vi "Frequency_current_field map_MFLI_PK_v4.0_measureXandY.vi"() -> ()   [LabVIEW 2016]
uses:
  <vilib>/Math Plots/2D Math Plots/2D Compass/2D Compass XCtrl/2D Compass.xctl
  <vilib>/Math Plots/2D Math Plots/2D Compass/2D Compass Datatype/2D Compass Datatype.lvclass
  Labview Drivers/MFLI/LabOneLabVIEW-22.02.26577/LabOneLabVIEW-22.02.26577/Zurich Instruments LabOne/Public/Configure/ziSetValueDouble.vi
  <vilib>/Math Plots/2D Math Plots/2D Compass/2D Compass Datatype/Public/Plot Helper (Vector).vi
  Labview Drivers/MFLI/LabOneLabVIEW-22.02.26577/LabOneLabVIEW-22.02.26577/Zurich Instruments LabOne/Public/Configure/ziGetValueDemodSampleEx.vi
  Labview Drivers/MFLI/LabOneLabVIEW-22.02.26577/LabOneLabVIEW-22.02.26577/Zurich Instruments LabOne/Zurich Instruments LabOne.lvlib
panel:
  in  "Measure Second Harmonic Current?":bool=TRUE
  in  "Number averaging (second harmonic)":i32=50
  in  "Autorange ON?":bool
  in  "Measure Second Harmonic Voltage?":bool
  in  "MFLI Current source/Voltage reader":string="DEV3647"
  out "data":dbl[](array[numeric])=[0.38999904300210686, 122.13037074970735, 6.972893577431705e-07, 1.2795166180217325e-05, 6.450568250497636e-11, 0.0, 170.15838700076765, 179.8047672609114, -20.097468935278, 0.0, 70441.803]
  in  "Number averaging (first harmonic)":i32=1
  in  "wait (ms) [Should be > TC]":u32=5000
  out "2D Compass":refnum<class "2D Plot Datatype.lvclass">[](xcontrol)
  in  "Step 3":dbl[](array[numeric])=[0.04, 0.04] min=-3000.0 max=3000.0 format="%.1e"
  in  "To 3":dbl[](array[numeric])=[7.0, -7.0] min=-3000.0 max=3000.0 format="%.1e"
  in  "From 3":dbl[](array[numeric])=[0.0, 0.0] min=-3000.0 max=3000.0 format="%.1e"
  in  "Tab Control":enum32{"Page 1", "Page 2"}(tab)=enum."Page 2"
  out "Iw vs Vw":cluster{dbl, "Field Reading":dbl}[](graph)=[{6.752718621134307e-13, "Field Reading"=6.081816034517228e-09}, {3.9639798477387415e-09, "Field Reading"=6.446162839710732e-08}, {7.973337710224394e-09, "Field Reading"=1.3070822529689762e-07}, {1.1980894320007212e-08, "Field Reading"=2.1301708498159723e-07}, {1.5990904057993272e-08, "Field Reading"=2.8268544133918733e-07}, {1.9996111650797034e-08, "Field Reading"=3.5482236477303006e-07}, {2.400534666117059e-08, "Field Reading"=4.2327567430694e-07}, {2.800722349467468e-08, "Field Reading"=5.024481108748963e-07}, {3.201355214200622e-08, "Field Reading"=5.73207701290961e-07}, {3.602886057924252e-08, "Field Reading"=6.408242032206597e-07}, {4.0029592079284544e-08, "Field Reading"=7.150994635609651e-07}, {4.4043549463955937e-08, "Field Reading"=7.890491387847592e-07}, {4.8050410980351376e-08, "Field Reading"=8.636898236498978e-07}, {5.205405189864272e-08, "Field Reading"=9.359032020670712e-07}, {5.6056170335994144e-08, "Field Reading"=1.0134208250064639e-06}, {6.006110040781738e-08, "Field Reading"=1.0801189896734763e-06}, {6.407650457950991e-08, "Field Reading"=1.157017799271746e-06}, {6.807679850147895e-08, "Field Reading"=1.223571908735428e-06}, {7.21023440572555e-08, "Field Reading"=1.300878249090366e-06}, {7.612142197841778e-08, "Field Reading"=1.3740376616836122e-06}, {8.013380677703043e-08, "Field Reading"=1.4497798169438424e-06}, {8.413258883874902e-08, "Field Reading"=1.5199655499746968e-06}, {8.81468182126121e-08, "Field Reading"=1.5948188164522483e-06}, {9.214947750799019e-08, "Field Reading"=1.6669947570028151e-06}, {9.61591330581471e-08, "Field Reading"=1.7421137383698782e-06}, {1.0016253832106813e-07, "Field Reading"=1.8098314979660362e-06}, {1.0417257692340365e-07, "Field Reading"=1.8855513250381588e-06}, {1.0818369532898691e-07, "Field Reading"=1.9618785093887747e-06}, {1.1218582132451216e-07, "Field Reading"=2.0348711393931705e-06}, {1.1619441564382123e-07, "Field Reading"=2.10788864479139e-06}, {1.2020719866139288e-07, "Field Reading"=2.183351428437738e-06}, {1.2421432089677758e-07, "Field Reading"=2.2548907316702294e-06}, {1.2821366558565993e-07, "Field Reading"=2.3242128448734923e-06}, {1.3222154670961958e-07, "Field Reading"=2.4006507162449404e-06}, {1.3623903792040753e-07, "Field Reading"=2.4756602824151876e-06}, {1.4024313259907697e-07, "Field Reading"=2.552042614165629e-06}, {1.442521785883789e-07, "Field Reading"=2.620144756978161e-06}, {1.4825805446265412e-07, "Field Reading"=2.692379499895667e-06}, {1.5226941875485597e-07, "Field Reading"=2.7663974907389294e-06}, {1.5627669910985748e-07, "Field Reading"=2.839358194975161e-06}, {1.6028888336617344e-07, "Field Reading"=2.911681627856578e-06}, {1.64302772644462e-07, "Field Reading"=2.9888815311636043e-06}, {1.6830688204588808e-07, "Field Reading"=3.057033036041899e-06}, {1.72312249131026e-07, "Field Reading"=3.134796277755431e-06}, {1.7632530452368395e-07, "Field Reading"=3.2066343708058573e-06}, {1.8034298753162188e-07, "Field Reading"=3.2795756506086883e-06}, {1.8433281290203653e-07, "Field Reading"=3.3535223874428235e-06}, {1.8834454582758565e-07, "Field Reading"=3.427737815687775e-06}, {1.923525886788216e-07, "Field Reading"=3.5037940525395852e-06}, {1.9636648414922318e-07, "Field Reading"=3.575940709860304e-06}, {2.003643068727201e-07, "Field Reading"=3.6476811261535922e-06}, {2.0438258512120876e-07, "Field Reading"=3.7191101089781536e-06}, {2.0839002189648273e-07, "Field Reading"=3.795291495640923e-06}, {2.124038020058244e-07, "Field Reading"=3.867976095996228e-06}, {2.164023667169985e-07, "Field Reading"=3.9392937163044255e-06}, {2.2042055698441663e-07, "Field Reading"=4.014886152002913e-06}, {2.2442432876248857e-07, "Field Reading"=4.088888686249118e-06}, {2.284312216677851e-07, "Field Reading"=4.162362043129873e-06}, {2.3244661758681178e-07, "Field Reading"=4.235758863815432e-06}, {2.3644759593726386e-07, "Field Reading"=4.312355387793181e-06}, {2.40459100592141e-07, "Field Reading"=4.3837197112583985e-06}, {2.444529691753868e-07, "Field Reading"=4.457438197792255e-06}, {2.484731479349489e-07, "Field Reading"=4.536782845780873e-06}, {2.524719528533667e-07, "Field Reading"=4.5990035451671585e-06}, {2.5649035151823195e-07, "Field Reading"=4.674219473122293e-06}, {2.6049079932691624e-07, "Field Reading"=4.754493036596978e-06}, {2.645024431202953e-07, "Field Reading"=4.8229123783948095e-06}, {2.685035511024019e-07, "Field Reading"=4.902907714190253e-06}, {2.7250559729734373e-07, "Field Reading"=4.973338061045356e-06}, {2.765088983761033e-07, "Field Reading"=5.0435466472495134e-06}, {2.8052562384174734e-07, "Field Reading"=5.122127663717767e-06}, {2.845332980147583e-07, "Field Reading"=5.1952956260170585e-06}, {2.8853853813904136e-07, "Field Reading"=5.276049411913597e-06}, {2.9255082029007556e-07, "Field Reading"=5.338393085315031e-06}, {2.965589694513312e-07, "Field Reading"=5.414829696556309e-06}, {3.005655236869771e-07, "Field Reading"=5.486743033872425e-06}, {3.0457127604346063e-07, "Field Reading"=5.561439221710705e-06}, {3.0857328583595214e-07, "Field Reading"=5.635709896350234e-06}, {3.125780613188083e-07, "Field Reading"=5.710622154466396e-06}, {3.1657800532807683e-07, "Field Reading"=5.7785483182008366e-06}, {3.205859793496837e-07, "Field Reading"=5.857257666587692e-06}, {3.2459851875999915e-07, "Field Reading"=5.933638774436689e-06}, {3.2861411834016656e-07, "Field Reading"=6.006913317833202e-06}, {3.326041181095403e-07, "Field Reading"=6.083532252465091e-06}, {3.366250625584465e-07, "Field Reading"=6.154442471014648e-06}, {3.406330536788778e-07, "Field Reading"=6.229292535120157e-06}, {3.4463787946499883e-07, "Field Reading"=6.298496219763628e-06}, {3.4864249001668815e-07, "Field Reading"=6.373935145038675e-06}, {3.5266166624564516e-07, "Field Reading"=6.451494387317105e-06}, {3.5666389193853506e-07, "Field Reading"=6.514138102733205e-06}, {3.606647597559832e-07, "Field Reading"=6.593143261943194e-06}, {3.646750692701237e-07, "Field Reading"=6.665398954773506e-06}, {3.686869138293502e-07, "Field Reading"=6.74274312075813e-06}, {3.726946403456541e-07, "Field Reading"=6.813468465941209e-06}, {3.7669898094509526e-07, "Field Reading"=6.8856155861323415e-06}, {3.80713112581362e-07, "Field Reading"=6.966944500326797e-06}, {3.8472237511467064e-07, "Field Reading"=7.042425427008974e-06}, {3.8873229351956887e-07, "Field Reading"=7.1114276716412805e-06}, {3.927256933734159e-07, "Field Reading"=7.187267238196006e-06}, {3.967382699755616e-07, "Field Reading"=7.255760952145238e-06}, {4.007403346966149e-07, "Field Reading"=7.332970273386945e-06}, {4.0474117306471594e-07, "Field Reading"=7.398287477833807e-06}, {4.0876584765236005e-07, "Field Reading"=7.481043329739446e-06}, {4.127782337495444e-07, "Field Reading"=7.561245791041404e-06}, {4.167710748588386e-07, "Field Reading"=7.625287150125578e-06}, {4.207843547855495e-07, "Field Reading"=7.69946278803481e-06}, {4.2478514945557536e-07, "Field Reading"=7.77262746884222e-06}, {4.2880134280692003e-07, "Field Reading"=7.852636002869716e-06}, {4.32792746566576e-07, "Field Reading"=7.920091802554008e-06}, {4.3680613506318253e-07, "Field Reading"=7.99498395075553e-06}, {4.4081431807847446e-07, "Field Reading"=8.073322022266602e-06}, {4.448169330741503e-07, "Field Reading"=8.141452378236027e-06}, {4.488206033855375e-07, "Field Reading"=8.215523961484074e-06}, {4.5283229725978943e-07, "Field Reading"=8.296738126475706e-06}, {4.5684372674779274e-07, "Field Reading"=8.36464717070889e-06}, {4.608385886916715e-07, "Field Reading"=8.435815670392521e-06}, {4.648372028608092e-07, "Field Reading"=8.50960183432341e-06}, {4.688434660258604e-07, "Field Reading"=8.583646136951763e-06}, {4.7284828197185846e-07, "Field Reading"=8.661893728175319e-06}, {4.768439287079396e-07, "Field Reading"=8.736479884477248e-06}, {4.808619754053666e-07, "Field Reading"=8.809133393554074e-06}, {4.848645388187712e-07, "Field Reading"=8.882270213481318e-06}, {4.888608773602841e-07, "Field Reading"=8.957131138329231e-06}, {4.928773928894314e-07, "Field Reading"=9.029727125247536e-06}, {4.9688603946784e-07, "Field Reading"=9.09868256245665e-06}, {5.008984812780072e-07, "Field Reading"=9.179684427963169e-06}, {5.049082694364706e-07, "Field Reading"=9.249396431237732e-06}, {5.089078867339119e-07, "Field Reading"=9.324815631609967e-06}, {5.129207792266292e-07, "Field Reading"=9.395502077706966e-06}, {5.16916821905768e-07, "Field Reading"=9.472861187304162e-06}, {5.209265519237412e-07, "Field Reading"=9.546361127234214e-06}, {5.249452832449703e-07, "Field Reading"=9.618642611519832e-06}, {5.289438730221308e-07, "Field Reading"=9.694146727945345e-06}, {5.329597666740567e-07, "Field Reading"=9.767514041008244e-06}, {5.36959974106049e-07, "Field Reading"=9.839237049373114e-06}, {5.409662739596735e-07, "Field Reading"=9.914717226759983e-06}, {5.449718528352936e-07, "Field Reading"=9.990606585930911e-06}, {5.489786573931961e-07, "Field Reading"=1.0068577997840325e-05}, {5.529795197615837e-07, "Field Reading"=1.0136510865604639e-05}, {5.569935375050876e-07, "Field Reading"=1.0204353143660428e-05}, {5.610099608578356e-07, "Field Reading"=1.0287332733542272e-05}, {5.650150940524591e-07, "Field Reading"=1.0364184451311051e-05}, {5.690251886958287e-07, "Field Reading"=1.0434862772017799e-05}, {5.730169395286551e-07, "Field Reading"=1.0508974657641133e-05}, {5.770317848841414e-07, "Field Reading"=1.058225379853519e-05}, {5.810402693058221e-07, "Field Reading"=1.0643951886158547e-05}, {5.850385166513102e-07, "Field Reading"=1.0725287037518511e-05}, {5.890559617454273e-07, "Field Reading"=1.0803765882597764e-05}, {5.930620244448425e-07, "Field Reading"=1.087588955313183e-05}, {5.970691912424186e-07, "Field Reading"=1.0955708857144528e-05}, {6.010636610044308e-07, "Field Reading"=1.1022087238492938e-05}, {6.050869253358961e-07, "Field Reading"=1.1092486372215814e-05}, {6.09091758211083e-07, "Field Reading"=1.1171170102501748e-05}, {6.131038344649093e-07, "Field Reading"=1.1245702001760147e-05}, {6.171179741498633e-07, "Field Reading"=1.1315855906438373e-05}, {6.211173983599906e-07, "Field Reading"=1.1398578240820748e-05}, {6.25124464451616e-07, "Field Reading"=1.1470196348734225e-05}, {6.291143503695416e-07, "Field Reading"=1.1539420089136223e-05}, {6.331521942370854e-07, "Field Reading"=1.1612792846117975e-05}, {6.371585234008393e-07, "Field Reading"=1.168916434048833e-05}, {6.411653272180744e-07, "Field Reading"=1.1765692996642987e-05}, {6.451832442213258e-07, "Field Reading"=1.1837901362754748e-05}, {6.491850515885537e-07, "Field Reading"=1.1909649783672709e-05}, {6.531930037237445e-07, "Field Reading"=1.198364650491436e-05}, {6.57186432677824e-07, "Field Reading"=1.2060179816420713e-05}, {6.611944104561734e-07, "Field Reading"=1.2123913771082415e-05}, {6.652137445236548e-07, "Field Reading"=1.2211051397225869e-05}, {6.692383358637068e-07, "Field Reading"=1.228412079260952e-05}, {6.732320428385544e-07, "Field Reading"=1.2349533947404962e-05}, {6.77225045428776e-07, "Field Reading"=1.2431989103460716e-05}, {6.812433375195916e-07, "Field Reading"=1.2506056808250104e-05}, {6.852323969852692e-07, "Field Reading"=1.2570407083013278e-05}, {6.892588291001929e-07, "Field Reading"=1.2642367874243355e-05}, {6.932649734064215e-07, "Field Reading"=1.272520742379873e-05}, {6.972796026622005e-07, "Field Reading"=1.2799370686555177e-05}, {3.695457990726968e-13, "Field Reading"=5.698071894479665e-09}, {3.9587514266942006e-09, "Field Reading"=6.824533699184529e-08}, {7.96951312709428e-09, "Field Reading"=1.3985866558682618e-07}, {1.1979948269645202e-08, "Field Reading"=2.0876330521373007e-07}, {1.5983895481099715e-08, "Field Reading"=2.8553830537874887e-07}, {1.999461838939512e-08, "Field Reading"=3.5439162282040604e-07}, {2.400475052994454e-08, "Field Reading"=4.298294578476292e-07}, {2.8008164339990668e-08, "Field Reading"=4.987382728457851e-07}, {3.2017033835969435e-08, "Field Reading"=5.688707826463316e-07}, {3.6024138533788023e-08, "Field Reading"=6.444474335860795e-07}, {4.0033084139702645e-08, "Field Reading"=7.195800417578632e-07}, {4.404046569235817e-08, "Field Reading"=7.927852549096227e-07}, {4.804030826522434e-08, "Field Reading"=8.629720258383935e-07}, {5.2053716184112815e-08, "Field Reading"=9.360625502405603e-07}, {5.605280909327427e-08, "Field Reading"=1.0125975343316225e-06}, {6.006067257344079e-08, "Field Reading"=1.0764321470005743e-06}, {6.406676809702357e-08, "Field Reading"=1.1588846026323697e-06}, {6.807860867321008e-08, "Field Reading"=1.2332259105577365e-06}, {7.210710309990868e-08, "Field Reading"=1.3038192588178447e-06}, {7.61215638566199e-08, "Field Reading"=1.377617098101442e-06}, {8.013214642451544e-08, "Field Reading"=1.452241236858506e-06}, {8.413063130992341e-08, "Field Reading"=1.5205875191624804e-06}, {8.814196552563718e-08, "Field Reading"=1.5973871888974442e-06}, {9.214185329913215e-08, "Field Reading"=1.6636245029512032e-06}, {9.614508769864244e-08, "Field Reading"=1.7505852312657933e-06}, {1.0015602426408757e-07, "Field Reading"=1.8159915918622937e-06}, {1.0416799861410451e-07, "Field Reading"=1.889798444386677e-06}, {1.0817850150530281e-07, "Field Reading"=1.9621860666582506e-06}, {1.1218636839353559e-07, "Field Reading"=2.037082818202477e-06}, {1.1618679588891763e-07, "Field Reading"=2.1122360696148114e-06}, {1.20206814334114e-07, "Field Reading"=2.1777435655423606e-06}, {1.2420841447754306e-07, "Field Reading"=2.255640179281544e-06}, {1.2821319899579289e-07, "Field Reading"=2.3312999651233155e-06}, {1.3222583172501857e-07, "Field Reading"=2.4024085147188928e-06}, {1.3623342017385734e-07, "Field Reading"=2.470034801634953e-06}, {1.4023759008988892e-07, "Field Reading"=2.542095290460891e-06}, {1.4424507010539416e-07, "Field Reading"=2.6170694941540647e-06}, {1.4825488632240412e-07, "Field Reading"=2.6910231312422564e-06}, {1.5226944571136413e-07, "Field Reading"=2.767609787104627e-06}, {1.5627380498979698e-07, "Field Reading"=2.836982731189964e-06}, {1.6028521355674098e-07, "Field Reading"=2.9124222293071654e-06}, {1.6429549429076714e-07, "Field Reading"=2.98472936879348e-06}, {1.6830459853200048e-07, "Field Reading"=3.0613950402695295e-06}, {1.7230366928244657e-07, "Field Reading"=3.1341415581016698e-06}, {1.763177572165781e-07, "Field Reading"=3.2064854067003242e-06}, {1.8032634203251206e-07, "Field Reading"=3.2845130790126582e-06}, {1.843385157463384e-07, "Field Reading"=3.3538281951650226e-06}, {1.883360416878448e-07, "Field Reading"=3.4263295581242788e-06}, {1.9235097490243074e-07, "Field Reading"=3.5074895309486576e-06}, {1.963587115606858e-07, "Field Reading"=3.5723242839209554e-06}, {2.0035576123493957e-07, "Field Reading"=3.6475948759770374e-06}, {2.0437128654225753e-07, "Field Reading"=3.7218891800187525e-06}, {2.0839327750961732e-07, "Field Reading"=3.7922256473378546e-06}, {2.1240028490422649e-07, "Field Reading"=3.872031784491173e-06}, {2.164061391970429e-07, "Field Reading"=3.945420127797786e-06}, {2.204174174016725e-07, "Field Reading"=4.021578337019413e-06}, {2.244213840752897e-07, "Field Reading"=4.092386623889813e-06}, {2.284271593682132e-07, "Field Reading"=4.166951249319548e-06}, {2.3242717177197805e-07, "Field Reading"=4.236549079746125e-06}, {2.364378821769146e-07, "Field Reading"=4.311334792355854e-06}, {2.404587274544687e-07, "Field Reading"=4.388619871276434e-06}, {2.4445827509569344e-07, "Field Reading"=4.458633334353797e-06}, {2.484639539614582e-07, "Field Reading"=4.53699551342188e-06}, {2.5247251325782825e-07, "Field Reading"=4.608124088996196e-06}, {2.564864821249374e-07, "Field Reading"=4.676182220931797e-06}, {2.604810430740118e-07, "Field Reading"=4.749533663063404e-06}, {2.644922890184137e-07, "Field Reading"=4.832174173068287e-06}, {2.685017817576427e-07, "Field Reading"=4.898860317406063e-06}, {2.7250814828756673e-07, "Field Reading"=4.975528351103424e-06}, {2.7651510514395105e-07, "Field Reading"=5.047764978603785e-06}, {2.8052364030662375e-07, "Field Reading"=5.121023562689988e-06}, {2.845325098385667e-07, "Field Reading"=5.191596520538841e-06}, {2.8852780990468735e-07, "Field Reading"=5.266104213036381e-06}, {2.9253698894593535e-07, "Field Reading"=5.339115119283014e-06}, {2.965481465083192e-07, "Field Reading"=5.4160485405172955e-06}, {3.005509495572527e-07, "Field Reading"=5.494915806924091e-06}, {3.045556885916384e-07, "Field Reading"=5.562080696404206e-06}, {3.0856645522803797e-07, "Field Reading"=5.640022217720643e-06}, {3.1257657708335385e-07, "Field Reading"=5.711968405659509e-06}, {3.165750585263558e-07, "Field Reading"=5.783886367669718e-06}, {3.205868903108242e-07, "Field Reading"=5.865148500569075e-06}, {3.2460314250582997e-07, "Field Reading"=5.932597590428266e-06}, {3.2861616400364176e-07, "Field Reading"=6.005949376746854e-06}, {3.3260995873295346e-07, "Field Reading"=6.077729052169175e-06}, {3.3660992509423754e-07, "Field Reading"=6.152365015910243e-06}, {3.406347123545983e-07, "Field Reading"=6.226174256027512e-06}, {3.446438482062892e-07, "Field Reading"=6.299362766035275e-06}, {3.4864186399793596e-07, "Field Reading"=6.37414832191692e-06}, {3.5265247503792236e-07, "Field Reading"=6.4456282419928234e-06}, {3.56665376184869e-07, "Field Reading"=6.529403005613757e-06}, {3.6066734451414065e-07, "Field Reading"=6.598974149679032e-06}, {3.646819848739686e-07, "Field Reading"=6.669921751490827e-06}, {3.68682217504304e-07, "Field Reading"=6.74306226885469e-06}, {3.727065021065556e-07, "Field Reading"=6.813830310377108e-06}, {3.767008614692342e-07, "Field Reading"=6.889393283775725e-06}, {3.807063218593253e-07, "Field Reading"=6.9638747325355745e-06}, {3.84719016492907e-07, "Field Reading"=7.04128753160004e-06}, {3.887276604305829e-07, "Field Reading"=7.105086495008707e-06}, {3.9272401348056196e-07, "Field Reading"=7.184782839715714e-06}, {3.9673291791571813e-07, "Field Reading"=7.256439856497261e-06}, {4.007442843832284e-07, "Field Reading"=7.333113887113307e-06}, {4.0474697892816316e-07, "Field Reading"=7.406217828105429e-06}, {4.0875677214397327e-07, "Field Reading"=7.480073316850151e-06}, {4.127648928978671e-07, "Field Reading"=7.555521781310909e-06}, {4.1677390804238657e-07, "Field Reading"=7.629965109442134e-06}, {4.207784398524056e-07, "Field Reading"=7.699214206031809e-06}, {4.2479118536657584e-07, "Field Reading"=7.777609218528186e-06}, {4.2879348216478443e-07, "Field Reading"=7.848748128930635e-06}, {4.3281368700915934e-07, "Field Reading"=7.927107003998515e-06}, {4.3679043785765377e-07, "Field Reading"=7.991439002710923e-06}, {4.408048794075155e-07, "Field Reading"=8.067457866553554e-06}, {4.4481269705169036e-07, "Field Reading"=8.144639903942311e-06}, {4.488200396041691e-07, "Field Reading"=8.214798069684028e-06}, {4.528261552426099e-07, "Field Reading"=8.288810559972375e-06}, {4.568249367581602e-07, "Field Reading"=8.362134306894896e-06}, {4.6083876371440633e-07, "Field Reading"=8.441314782601667e-06}, {4.6484674569200007e-07, "Field Reading"=8.516255633827248e-06}, {4.6886211987917445e-07, "Field Reading"=8.585900603542732e-06}, {4.728744132518244e-07, "Field Reading"=8.660223005475944e-06}, {4.768710286573309e-07, "Field Reading"=8.734395533820769e-06}, {4.808789492496296e-07, "Field Reading"=8.81077402330044e-06}, {4.84900141033635e-07, "Field Reading"=8.88221335148442e-06}, {4.889096292480101e-07, "Field Reading"=8.952780895721028e-06}, {4.929011448030727e-07, "Field Reading"=9.023233785652485e-06}, {4.96914094104685e-07, "Field Reading"=9.104837016112909e-06}, {5.009124658723474e-07, "Field Reading"=9.176498231786628e-06}, {5.049277646516033e-07, "Field Reading"=9.249998779045577e-06}, {5.089242736925264e-07, "Field Reading"=9.323919830596103e-06}, {5.129328196325962e-07, "Field Reading"=9.393459654395195e-06}, {5.16938938636249e-07, "Field Reading"=9.47134583847599e-06}, {5.209582762725067e-07, "Field Reading"=9.546837597673096e-06}, {5.249599054021532e-07, "Field Reading"=9.618382737867968e-06}, {5.289653219925673e-07, "Field Reading"=9.694529837036145e-06}, {5.329687909235363e-07, "Field Reading"=9.76751027295797e-06}, {5.369619247055903e-07, "Field Reading"=9.844620993541572e-06}, {5.40969967063774e-07, "Field Reading"=9.912999800724708e-06}, {5.449778733989274e-07, "Field Reading"=9.990301579757168e-06}, {5.489887919647749e-07, "Field Reading"=1.0064592865440964e-05}, {5.529916068346236e-07, "Field Reading"=1.0142889568006644e-05}, {5.56988870365852e-07, "Field Reading"=1.021472085789113e-05}, {5.610052420776777e-07, "Field Reading"=1.0289674029122719e-05}, {5.650190658830066e-07, "Field Reading"=1.0360405759120638e-05}, {5.690190702763405e-07, "Field Reading"=1.0435454384407978e-05}, {5.730444454840748e-07, "Field Reading"=1.051298872134457e-05}, {5.770597664108027e-07, "Field Reading"=1.0579031486891604e-05}, {5.810602653692694e-07, "Field Reading"=1.0652944257386492e-05}, {5.850728145256359e-07, "Field Reading"=1.0726243307849132e-05}, {5.890767670181646e-07, "Field Reading"=1.0806947934543218e-05}, {5.930767090913838e-07, "Field Reading"=1.0882796022214024e-05}, {5.970839166377572e-07, "Field Reading"=1.0954573224921726e-05}, {6.011068573945384e-07, "Field Reading"=1.102260076791975e-05}, {6.051002836487515e-07, "Field Reading"=1.1098742423853433e-05}, {6.091153782577642e-07, "Field Reading"=1.1170709784497336e-05}, {6.131153170489284e-07, "Field Reading"=1.1251955700466336e-05}, {6.171206045524325e-07, "Field Reading"=1.1323281210948316e-05}, {6.21125067983006e-07, "Field Reading"=1.1400015059159992e-05}, {6.251268851331833e-07, "Field Reading"=1.1465098896193353e-05}, {6.291438341148671e-07, "Field Reading"=1.1540414658402066e-05}, {6.33130907845599e-07, "Field Reading"=1.1614826739965938e-05}, {6.371470053501204e-07, "Field Reading"=1.1689446616607722e-05}, {6.411561580168332e-07, "Field Reading"=1.1763747227943706e-05}, {6.451858613647945e-07, "Field Reading"=1.1833126732492007e-05}, {6.491750497259894e-07, "Field Reading"=1.1909692915691624e-05}, {6.531963349907788e-07, "Field Reading"=1.198589421633311e-05}, {6.57207107516709e-07, "Field Reading"=1.2059265376888092e-05}, {6.612002662512429e-07, "Field Reading"=1.2131046148000714e-05}, {6.652059118331257e-07, "Field Reading"=1.220693579151733e-05}, {6.692193621767105e-07, "Field Reading"=1.22842018338008e-05}, {6.732075867086699e-07, "Field Reading"=1.2354259434976681e-05}, {6.772319470513882e-07, "Field Reading"=1.242573840875969e-05}, {6.812475180349191e-07, "Field Reading"=1.251079414204885e-05}, {6.852374483111342e-07, "Field Reading"=1.257628484636858e-05}, {6.892677466242672e-07, "Field Reading"=1.2653903437863818e-05}, {6.932781230420922e-07, "Field Reading"=1.2727229374328647e-05}, {6.972893577431705e-07, "Field Reading"=1.2795166180217325e-05}]
  out "I2w (A)":dbl=6.450568250497636e-11
  out "V2w (V)":dbl
  out "Iw (A)":dbl=6.972893577431705e-07
  out "Iw_phase (deg)":dbl=170.15838700076765 format="%#_13g"
  out "Vw (V)":dbl=1.2795166180217325e-05
  out "Vw_phase (deg)":dbl=179.8047672609114 format="%#_13g"
  out "Set Voltage(V)":dbl=-9.84292639411675 format="%#_13g"
  out "Time(s)":dbl=70441.803 format="%#_13g"
  out "I2w_phase (deg)":dbl=-20.097468935278 format="%#_13g"
  out "V2w_phase (deg)":dbl format="%#_13g"
  out "I2w vs Iw":cluster{dbl, "Field Reading":dbl}[](graph)=[{6.752718621134307e-13, "Field Reading"=2.540215775246723e-13}, {3.9639798477387415e-09, "Field Reading"=2.6121334770459845e-12}, {7.973337710224394e-09, "Field Reading"=2.0377945378656124e-12}, {1.1980894320007212e-08, "Field Reading"=2.778071667579133e-12}, {1.5990904057993272e-08, "Field Reading"=2.498846157025503e-12}, {1.9996111650797034e-08, "Field Reading"=1.8837580878055735e-12}, {2.400534666117059e-08, "Field Reading"=2.9217257909799205e-12}, {2.800722349467468e-08, "Field Reading"=1.2408163114046102e-12}, {3.201355214200622e-08, "Field Reading"=1.7629255187333967e-12}, {3.602886057924252e-08, "Field Reading"=2.018708147155936e-12}, {4.0029592079284544e-08, "Field Reading"=7.886162039170557e-13}, {4.4043549463955937e-08, "Field Reading"=2.8246552394199483e-12}, {4.8050410980351376e-08, "Field Reading"=1.2235994978906469e-12}, {5.205405189864272e-08, "Field Reading"=2.644211497717227e-12}, {5.6056170335994144e-08, "Field Reading"=1.3684766141680678e-12}, {6.006110040781738e-08, "Field Reading"=1.1836658755940086e-12}, {6.407650457950991e-08, "Field Reading"=2.235459202881915e-12}, {6.807679850147895e-08, "Field Reading"=9.729688955419961e-13}, {7.21023440572555e-08, "Field Reading"=1.1814396345161887e-11}, {7.612142197841778e-08, "Field Reading"=1.1785466767345847e-11}, {8.013380677703043e-08, "Field Reading"=1.2035102266329501e-11}, {8.413258883874902e-08, "Field Reading"=1.1787630410946756e-11}, {8.81468182126121e-08, "Field Reading"=9.129742332407166e-12}, {9.214947750799019e-08, "Field Reading"=1.033546784505753e-11}, {9.61591330581471e-08, "Field Reading"=1.2123940555621325e-11}, {1.0016253832106813e-07, "Field Reading"=9.689037476398541e-12}, {1.0417257692340365e-07, "Field Reading"=1.080083760883203e-11}, {1.0818369532898691e-07, "Field Reading"=1.2497874907576727e-11}, {1.1218582132451216e-07, "Field Reading"=1.4665030971620474e-11}, {1.1619441564382123e-07, "Field Reading"=1.2342125070206615e-11}, {1.2020719866139288e-07, "Field Reading"=1.616203149927857e-11}, {1.2421432089677758e-07, "Field Reading"=1.2851640441157552e-11}, {1.2821366558565993e-07, "Field Reading"=1.5896882924367085e-11}, {1.3222154670961958e-07, "Field Reading"=1.4119144506488629e-11}, {1.3623903792040753e-07, "Field Reading"=1.250388596871486e-11}, {1.4024313259907697e-07, "Field Reading"=1.4775256013385735e-11}, {1.442521785883789e-07, "Field Reading"=1.4672116340031205e-11}, {1.4825805446265412e-07, "Field Reading"=1.4021899019250218e-11}, {1.5226941875485597e-07, "Field Reading"=1.4698447608535105e-11}, {1.5627669910985748e-07, "Field Reading"=1.4645581087440724e-11}, {1.6028888336617344e-07, "Field Reading"=1.553378665550328e-11}, {1.64302772644462e-07, "Field Reading"=1.4779248598863672e-11}, {1.6830688204588808e-07, "Field Reading"=1.543707856894362e-11}, {1.72312249131026e-07, "Field Reading"=1.519949802066083e-11}, {1.7632530452368395e-07, "Field Reading"=1.5743715585473236e-11}, {1.8034298753162188e-07, "Field Reading"=1.4207409174203727e-11}, {1.8433281290203653e-07, "Field Reading"=1.6044432054311044e-11}, {1.8834454582758565e-07, "Field Reading"=1.6002816819122775e-11}, {1.923525886788216e-07, "Field Reading"=2.0174419803341724e-11}, {1.9636648414922318e-07, "Field Reading"=2.059968665438357e-11}, {2.003643068727201e-07, "Field Reading"=2.016164350039611e-11}, {2.0438258512120876e-07, "Field Reading"=2.3667687802935574e-11}, {2.0839002189648273e-07, "Field Reading"=2.1856416542193945e-11}, {2.124038020058244e-07, "Field Reading"=2.5654034396396907e-11}, {2.164023667169985e-07, "Field Reading"=2.2994401791125607e-11}, {2.2042055698441663e-07, "Field Reading"=2.266592088694829e-11}, {2.2442432876248857e-07, "Field Reading"=2.440238662218269e-11}, {2.284312216677851e-07, "Field Reading"=2.5566886630157963e-11}, {2.3244661758681178e-07, "Field Reading"=2.890025645099675e-11}, {2.3644759593726386e-07, "Field Reading"=2.8182570348539977e-11}, {2.40459100592141e-07, "Field Reading"=2.928977666771924e-11}, {2.444529691753868e-07, "Field Reading"=3.066958341298326e-11}, {2.484731479349489e-07, "Field Reading"=3.209625154731619e-11}, {2.524719528533667e-07, "Field Reading"=3.264451552248229e-11}, {2.5649035151823195e-07, "Field Reading"=3.318956535231248e-11}, {2.6049079932691624e-07, "Field Reading"=3.37335010932016e-11}, {2.645024431202953e-07, "Field Reading"=3.0763102231648744e-11}, {2.685035511024019e-07, "Field Reading"=3.418658009474822e-11}, {2.7250559729734373e-07, "Field Reading"=3.5796418085787905e-11}, {2.765088983761033e-07, "Field Reading"=3.4815474973541285e-11}, {2.8052562384174734e-07, "Field Reading"=3.6164532600325935e-11}, {2.845332980147583e-07, "Field Reading"=3.967574463601413e-11}, {2.8853853813904136e-07, "Field Reading"=4.1219209656416e-11}, {2.9255082029007556e-07, "Field Reading"=4.095310840833821e-11}, {2.965589694513312e-07, "Field Reading"=4.0410146332783684e-11}, {3.005655236869771e-07, "Field Reading"=3.820479698209618e-11}, {3.0457127604346063e-07, "Field Reading"=4.2137836009754024e-11}, {3.0857328583595214e-07, "Field Reading"=3.9451625172654855e-11}, {3.125780613188083e-07, "Field Reading"=4.2371481330199476e-11}, {3.1657800532807683e-07, "Field Reading"=3.8881852757914235e-11}, {3.205859793496837e-07, "Field Reading"=3.771658107955753e-11}, {3.2459851875999915e-07, "Field Reading"=4.156223942591132e-11}, {3.2861411834016656e-07, "Field Reading"=3.729691749797255e-11}, {3.326041181095403e-07, "Field Reading"=3.818853589427644e-11}, {3.366250625584465e-07, "Field Reading"=3.867563543286446e-11}, {3.406330536788778e-07, "Field Reading"=4.0896864114161576e-11}, {3.4463787946499883e-07, "Field Reading"=4.049615787642101e-11}, {3.4864249001668815e-07, "Field Reading"=4.109707653892744e-11}, {3.5266166624564516e-07, "Field Reading"=3.6936103946973474e-11}, {3.5666389193853506e-07, "Field Reading"=3.9768558666395626e-11}, {3.606647597559832e-07, "Field Reading"=3.972307596471419e-11}, {3.646750692701237e-07, "Field Reading"=4.3807969619634275e-11}, {3.686869138293502e-07, "Field Reading"=4.241465760875651e-11}, {3.726946403456541e-07, "Field Reading"=4.333193505611894e-11}, {3.7669898094509526e-07, "Field Reading"=4.395923375273165e-11}, {3.80713112581362e-07, "Field Reading"=4.1158201011650476e-11}, {3.8472237511467064e-07, "Field Reading"=4.599634818218701e-11}, {3.8873229351956887e-07, "Field Reading"=4.4910724411118646e-11}, {3.927256933734159e-07, "Field Reading"=4.442976934059301e-11}, {3.967382699755616e-07, "Field Reading"=4.1494924497488085e-11}, {4.007403346966149e-07, "Field Reading"=4.327928671432316e-11}, {4.0474117306471594e-07, "Field Reading"=4.446850731516231e-11}, {4.0876584765236005e-07, "Field Reading"=4.7651102924287676e-11}, {4.127782337495444e-07, "Field Reading"=4.723442322285639e-11}, {4.167710748588386e-07, "Field Reading"=4.806634095914595e-11}, {4.207843547855495e-07, "Field Reading"=4.86904396373397e-11}, {4.2478514945557536e-07, "Field Reading"=4.941079980687742e-11}, {4.2880134280692003e-07, "Field Reading"=5.1576537234183364e-11}, {4.32792746566576e-07, "Field Reading"=5.0784095230428863e-11}, {4.3680613506318253e-07, "Field Reading"=5.3128892662127496e-11}, {4.4081431807847446e-07, "Field Reading"=5.155216721523001e-11}, {4.448169330741503e-07, "Field Reading"=5.105613828796419e-11}, {4.488206033855375e-07, "Field Reading"=5.226617929286254e-11}, {4.5283229725978943e-07, "Field Reading"=5.230436353459349e-11}, {4.5684372674779274e-07, "Field Reading"=5.050267037525422e-11}, {4.608385886916715e-07, "Field Reading"=4.84499271575798e-11}, {4.648372028608092e-07, "Field Reading"=5.0190924304783066e-11}, {4.688434660258604e-07, "Field Reading"=4.8448919752355426e-11}, {4.7284828197185846e-07, "Field Reading"=5.0993456513791535e-11}, {4.768439287079396e-07, "Field Reading"=5.017036670880965e-11}, {4.808619754053666e-07, "Field Reading"=5.325372655862345e-11}, {4.848645388187712e-07, "Field Reading"=5.3656986374214387e-11}, {4.888608773602841e-07, "Field Reading"=5.415062023945687e-11}, {4.928773928894314e-07, "Field Reading"=5.125431277495083e-11}, {4.9688603946784e-07, "Field Reading"=5.20620903173094e-11}, {5.008984812780072e-07, "Field Reading"=5.200329148338377e-11}, {5.049082694364706e-07, "Field Reading"=5.5944855456576576e-11}, {5.089078867339119e-07, "Field Reading"=5.559808794958296e-11}, {5.129207792266292e-07, "Field Reading"=5.3286662644534903e-11}, {5.16916821905768e-07, "Field Reading"=5.498606317557074e-11}, {5.209265519237412e-07, "Field Reading"=5.271909693376304e-11}, {5.249452832449703e-07, "Field Reading"=5.5509562837912806e-11}, {5.289438730221308e-07, "Field Reading"=5.4232980137627814e-11}, {5.329597666740567e-07, "Field Reading"=5.546771331901801e-11}, {5.36959974106049e-07, "Field Reading"=5.247671999342142e-11}, {5.409662739596735e-07, "Field Reading"=5.350919505243116e-11}, {5.449718528352936e-07, "Field Reading"=5.507408335848158e-11}, {5.489786573931961e-07, "Field Reading"=5.394514289016507e-11}, {5.529795197615837e-07, "Field Reading"=5.416509011512546e-11}, {5.569935375050876e-07, "Field Reading"=5.73465618608679e-11}, {5.610099608578356e-07, "Field Reading"=5.930803544847915e-11}, {5.650150940524591e-07, "Field Reading"=6.005414940478683e-11}, {5.690251886958287e-07, "Field Reading"=5.888737721954652e-11}, {5.730169395286551e-07, "Field Reading"=6.077411503763882e-11}, {5.770317848841414e-07, "Field Reading"=6.107877071768294e-11}, {5.810402693058221e-07, "Field Reading"=5.900724881515841e-11}, {5.850385166513102e-07, "Field Reading"=6.006440069880428e-11}, {5.890559617454273e-07, "Field Reading"=5.91486657994636e-11}, {5.930620244448425e-07, "Field Reading"=6.200190538257744e-11}, {5.970691912424186e-07, "Field Reading"=6.376389691530029e-11}, {6.010636610044308e-07, "Field Reading"=6.568419928169567e-11}, {6.050869253358961e-07, "Field Reading"=6.646824219614154e-11}, {6.09091758211083e-07, "Field Reading"=6.562652637844236e-11}, {6.131038344649093e-07, "Field Reading"=6.43058326727766e-11}, {6.171179741498633e-07, "Field Reading"=6.568558396814543e-11}, {6.211173983599906e-07, "Field Reading"=6.768436991877683e-11}, {6.25124464451616e-07, "Field Reading"=6.756103006652947e-11}, {6.291143503695416e-07, "Field Reading"=6.820302809524011e-11}, {6.331521942370854e-07, "Field Reading"=6.694996980417711e-11}, {6.371585234008393e-07, "Field Reading"=6.519799519752896e-11}, {6.411653272180744e-07, "Field Reading"=6.613374278434862e-11}, {6.451832442213258e-07, "Field Reading"=6.796003831239519e-11}, {6.491850515885537e-07, "Field Reading"=6.710962755139632e-11}, {6.531930037237445e-07, "Field Reading"=6.734378786394395e-11}, {6.57186432677824e-07, "Field Reading"=6.677330526833857e-11}, {6.611944104561734e-07, "Field Reading"=6.674662242254714e-11}, {6.652137445236548e-07, "Field Reading"=6.951367305557199e-11}, {6.692383358637068e-07, "Field Reading"=7.056981059966933e-11}, {6.732320428385544e-07, "Field Reading"=7.013612722864493e-11}, {6.77225045428776e-07, "Field Reading"=7.016545459975179e-11}, {6.812433375195916e-07, "Field Reading"=6.871880309362113e-11}, {6.852323969852692e-07, "Field Reading"=6.829047114108872e-11}, {6.892588291001929e-07, "Field Reading"=6.483165357707174e-11}, {6.932649734064215e-07, "Field Reading"=6.490006655716477e-11}, {6.972796026622005e-07, "Field Reading"=6.422401070609759e-11}, {3.695457990726968e-13, "Field Reading"=2.5282771557741105e-13}, {3.9587514266942006e-09, "Field Reading"=1.5930535501026506e-12}, {7.96951312709428e-09, "Field Reading"=2.8010787419509677e-12}, {1.1979948269645202e-08, "Field Reading"=2.013426834849837e-12}, {1.5983895481099715e-08, "Field Reading"=1.829543393434864e-12}, {1.999461838939512e-08, "Field Reading"=3.066066372911442e-12}, {2.400475052994454e-08, "Field Reading"=1.5706011088297255e-12}, {2.8008164339990668e-08, "Field Reading"=3.6665461606118e-12}, {3.2017033835969435e-08, "Field Reading"=2.237745011419964e-12}, {3.6024138533788023e-08, "Field Reading"=1.1721437631620448e-12}, {4.0033084139702645e-08, "Field Reading"=2.0262995104221244e-12}, {4.404046569235817e-08, "Field Reading"=3.664943475534297e-12}, {4.804030826522434e-08, "Field Reading"=2.263797066505037e-12}, {5.2053716184112815e-08, "Field Reading"=2.620818120649302e-12}, {5.605280909327427e-08, "Field Reading"=2.318384645557775e-12}, {6.006067257344079e-08, "Field Reading"=1.9418907259098453e-12}, {6.406676809702357e-08, "Field Reading"=2.531394132444377e-12}, {6.807860867321008e-08, "Field Reading"=1.567379129176001e-12}, {7.210710309990868e-08, "Field Reading"=1.0071141601975999e-11}, {7.61215638566199e-08, "Field Reading"=9.7246564671276e-12}, {8.013214642451544e-08, "Field Reading"=8.901859561486112e-12}, {8.413063130992341e-08, "Field Reading"=8.694430732977649e-12}, {8.814196552563718e-08, "Field Reading"=1.2309012341618928e-11}, {9.214185329913215e-08, "Field Reading"=1.2771534835221438e-11}, {9.614508769864244e-08, "Field Reading"=1.3247622019980793e-11}, {1.0015602426408757e-07, "Field Reading"=1.1623885984399354e-11}, {1.0416799861410451e-07, "Field Reading"=1.0960532276840816e-11}, {1.0817850150530281e-07, "Field Reading"=1.177907035266872e-11}, {1.1218636839353559e-07, "Field Reading"=1.4879678755840352e-11}, {1.1618679588891763e-07, "Field Reading"=1.5184060031636686e-11}, {1.20206814334114e-07, "Field Reading"=1.4358689089879189e-11}, {1.2420841447754306e-07, "Field Reading"=1.6463444299038886e-11}, {1.2821319899579289e-07, "Field Reading"=1.3332194594148655e-11}, {1.3222583172501857e-07, "Field Reading"=1.691280787353132e-11}, {1.3623342017385734e-07, "Field Reading"=1.478275840209281e-11}, {1.4023759008988892e-07, "Field Reading"=1.424375001618506e-11}, {1.4424507010539416e-07, "Field Reading"=1.4256112803461382e-11}, {1.4825488632240412e-07, "Field Reading"=1.4333770233563216e-11}, {1.5226944571136413e-07, "Field Reading"=1.2888064058912636e-11}, {1.5627380498979698e-07, "Field Reading"=1.0486184893392225e-11}, {1.6028521355674098e-07, "Field Reading"=1.1700279364616469e-11}, {1.6429549429076714e-07, "Field Reading"=1.0998345543133605e-11}, {1.6830459853200048e-07, "Field Reading"=1.2087743463677898e-11}, {1.7230366928244657e-07, "Field Reading"=1.3471449267382825e-11}, {1.763177572165781e-07, "Field Reading"=1.608972699679182e-11}, {1.8032634203251206e-07, "Field Reading"=1.7305910558522267e-11}, {1.843385157463384e-07, "Field Reading"=1.8368738005846515e-11}, {1.883360416878448e-07, "Field Reading"=1.9289506796775354e-11}, {1.9235097490243074e-07, "Field Reading"=1.9779973910331214e-11}, {1.963587115606858e-07, "Field Reading"=1.8126979945707045e-11}, {2.0035576123493957e-07, "Field Reading"=2.1452009833031672e-11}, {2.0437128654225753e-07, "Field Reading"=2.2998721643182e-11}, {2.0839327750961732e-07, "Field Reading"=2.1212307651756744e-11}, {2.1240028490422649e-07, "Field Reading"=2.2875441587449862e-11}, {2.164061391970429e-07, "Field Reading"=2.3773098810818826e-11}, {2.204174174016725e-07, "Field Reading"=2.7512188257361405e-11}, {2.244213840752897e-07, "Field Reading"=2.3892096852057306e-11}, {2.284271593682132e-07, "Field Reading"=2.699449181851823e-11}, {2.3242717177197805e-07, "Field Reading"=2.909431702211742e-11}, {2.364378821769146e-07, "Field Reading"=2.8973407441934445e-11}, {2.404587274544687e-07, "Field Reading"=2.7884583200848478e-11}, {2.4445827509569344e-07, "Field Reading"=3.027143193005267e-11}, {2.484639539614582e-07, "Field Reading"=3.1564504304575715e-11}, {2.5247251325782825e-07, "Field Reading"=2.9237575937923634e-11}, {2.564864821249374e-07, "Field Reading"=3.053670669953717e-11}, {2.604810430740118e-07, "Field Reading"=3.202430697005556e-11}, {2.644922890184137e-07, "Field Reading"=3.46554090746098e-11}, {2.685017817576427e-07, "Field Reading"=3.578845693699961e-11}, {2.7250814828756673e-07, "Field Reading"=3.7647775293476866e-11}, {2.7651510514395105e-07, "Field Reading"=3.5647085806780566e-11}, {2.8052364030662375e-07, "Field Reading"=3.656104758307045e-11}, {2.845325098385667e-07, "Field Reading"=3.813337986367964e-11}, {2.8852780990468735e-07, "Field Reading"=3.787286335856111e-11}, {2.9253698894593535e-07, "Field Reading"=3.824108014196267e-11}, {2.965481465083192e-07, "Field Reading"=4.132073204569839e-11}, {3.005509495572527e-07, "Field Reading"=4.2408680649944874e-11}, {3.045556885916384e-07, "Field Reading"=4.043608416368307e-11}, {3.0856645522803797e-07, "Field Reading"=4.378766502806668e-11}, {3.1257657708335385e-07, "Field Reading"=4.23446865354141e-11}, {3.165750585263558e-07, "Field Reading"=4.084687863264775e-11}, {3.205868903108242e-07, "Field Reading"=3.77712019884902e-11}, {3.2460314250582997e-07, "Field Reading"=3.8839688695298754e-11}, {3.2861616400364176e-07, "Field Reading"=3.9055940958325796e-11}, {3.3260995873295346e-07, "Field Reading"=4.136158645127124e-11}, {3.3660992509423754e-07, "Field Reading"=3.9915508760910296e-11}, {3.406347123545983e-07, "Field Reading"=4.125702084595111e-11}, {3.446438482062892e-07, "Field Reading"=4.074788836784656e-11}, {3.4864186399793596e-07, "Field Reading"=4.094992368976711e-11}, {3.5265247503792236e-07, "Field Reading"=3.868708943255324e-11}, {3.56665376184869e-07, "Field Reading"=4.103221476082204e-11}, {3.6066734451414065e-07, "Field Reading"=4.1234657494615655e-11}, {3.646819848739686e-07, "Field Reading"=4.260268639569677e-11}, {3.68682217504304e-07, "Field Reading"=4.240946718456471e-11}, {3.727065021065556e-07, "Field Reading"=4.3519965995171096e-11}, {3.767008614692342e-07, "Field Reading"=4.312434943636139e-11}, {3.807063218593253e-07, "Field Reading"=4.3130546030337724e-11}, {3.84719016492907e-07, "Field Reading"=4.008661675930759e-11}, {3.887276604305829e-07, "Field Reading"=4.221198007949393e-11}, {3.9272401348056196e-07, "Field Reading"=4.293936651182658e-11}, {3.9673291791571813e-07, "Field Reading"=4.623167191553964e-11}, {4.007442843832284e-07, "Field Reading"=4.5708175331670406e-11}, {4.0474697892816316e-07, "Field Reading"=4.6507344105935516e-11}, {4.0875677214397327e-07, "Field Reading"=4.6580875212270724e-11}, {4.127648928978671e-07, "Field Reading"=4.535138996722086e-11}, {4.1677390804238657e-07, "Field Reading"=4.5671496639393876e-11}, {4.207784398524056e-07, "Field Reading"=4.5770496014952985e-11}, {4.2479118536657584e-07, "Field Reading"=4.609142706204921e-11}, {4.2879348216478443e-07, "Field Reading"=4.733321843144122e-11}, {4.3281368700915934e-07, "Field Reading"=5.131715035553229e-11}, {4.3679043785765377e-07, "Field Reading"=5.323776363782982e-11}, {4.408048794075155e-07, "Field Reading"=5.20746578553526e-11}, {4.4481269705169036e-07, "Field Reading"=5.094516991074002e-11}, {4.488200396041691e-07, "Field Reading"=5.124597491329243e-11}, {4.528261552426099e-07, "Field Reading"=5.0694648259650356e-11}, {4.568249367581602e-07, "Field Reading"=5.21182348591489e-11}, {4.6083876371440633e-07, "Field Reading"=5.264139350935497e-11}, {4.6484674569200007e-07, "Field Reading"=4.984891293279687e-11}, {4.6886211987917445e-07, "Field Reading"=5.200959708629815e-11}, {4.728744132518244e-07, "Field Reading"=5.2887129747821636e-11}, {4.768710286573309e-07, "Field Reading"=5.3139990203683924e-11}, {4.808789492496296e-07, "Field Reading"=5.274328640383689e-11}, {4.84900141033635e-07, "Field Reading"=5.10394187848172e-11}, {4.889096292480101e-07, "Field Reading"=5.116674902217948e-11}, {4.929011448030727e-07, "Field Reading"=5.129311458492361e-11}, {4.96914094104685e-07, "Field Reading"=5.453118140549034e-11}, {5.009124658723474e-07, "Field Reading"=5.5317619441512025e-11}, {5.049277646516033e-07, "Field Reading"=5.4160712141388186e-11}, {5.089242736925264e-07, "Field Reading"=5.254562653859669e-11}, {5.129328196325962e-07, "Field Reading"=5.0589330539100945e-11}, {5.16938938636249e-07, "Field Reading"=5.403132441467029e-11}, {5.209582762725067e-07, "Field Reading"=5.161295249804235e-11}, {5.249599054021532e-07, "Field Reading"=5.140484581442028e-11}, {5.289653219925673e-07, "Field Reading"=5.310231597481294e-11}, {5.329687909235363e-07, "Field Reading"=5.6550392801717196e-11}, {5.369619247055903e-07, "Field Reading"=5.5442567728589046e-11}, {5.40969967063774e-07, "Field Reading"=5.496185734017828e-11}, {5.449778733989274e-07, "Field Reading"=5.746765226674961e-11}, {5.489887919647749e-07, "Field Reading"=5.7391109065635136e-11}, {5.529916068346236e-07, "Field Reading"=5.8103278479543546e-11}, {5.56988870365852e-07, "Field Reading"=5.765234035640036e-11}, {5.610052420776777e-07, "Field Reading"=5.760578045335417e-11}, {5.650190658830066e-07, "Field Reading"=5.583399297292977e-11}, {5.690190702763405e-07, "Field Reading"=5.7413386199988124e-11}, {5.730444454840748e-07, "Field Reading"=5.965623799055868e-11}, {5.770597664108027e-07, "Field Reading"=5.803920845830859e-11}, {5.810602653692694e-07, "Field Reading"=5.866732708139203e-11}, {5.850728145256359e-07, "Field Reading"=6.220428671391128e-11}, {5.890767670181646e-07, "Field Reading"=6.28457191652954e-11}, {5.930767090913838e-07, "Field Reading"=6.246047345077204e-11}, {5.970839166377572e-07, "Field Reading"=6.477595792134802e-11}, {6.011068573945384e-07, "Field Reading"=6.46726343069814e-11}, {6.051002836487515e-07, "Field Reading"=6.381069130657024e-11}, {6.091153782577642e-07, "Field Reading"=6.155997746024924e-11}, {6.131153170489284e-07, "Field Reading"=6.378432601235624e-11}, {6.171206045524325e-07, "Field Reading"=6.539002976056167e-11}, {6.21125067983006e-07, "Field Reading"=6.748621349202427e-11}, {6.251268851331833e-07, "Field Reading"=6.784349375094177e-11}, {6.291438341148671e-07, "Field Reading"=6.728069780676202e-11}, {6.33130907845599e-07, "Field Reading"=6.671980944956575e-11}, {6.371470053501204e-07, "Field Reading"=6.853978819520523e-11}, {6.411561580168332e-07, "Field Reading"=6.679258842188276e-11}, {6.451858613647945e-07, "Field Reading"=6.615636376498311e-11}, {6.491750497259894e-07, "Field Reading"=6.894322854010631e-11}, {6.531963349907788e-07, "Field Reading"=6.683473570332554e-11}, {6.57207107516709e-07, "Field Reading"=6.70014765968252e-11}, {6.612002662512429e-07, "Field Reading"=6.810761036318809e-11}, {6.652059118331257e-07, "Field Reading"=6.713753432347388e-11}, {6.692193621767105e-07, "Field Reading"=6.625772619668147e-11}, {6.732075867086699e-07, "Field Reading"=6.884905694478715e-11}, {6.772319470513882e-07, "Field Reading"=6.841461144489658e-11}, {6.812475180349191e-07, "Field Reading"=6.522473456669023e-11}, {6.852374483111342e-07, "Field Reading"=6.933465888948014e-11}, {6.892677466242672e-07, "Field Reading"=6.664557132943735e-11}, {6.932781230420922e-07, "Field Reading"=6.565116809569013e-11}, {6.972893577431705e-07, "Field Reading"=6.450568250497636e-11}]
  out "Magnetic Field Vector Angle":dbl=122.13037074970735 format="%#_13g"
  out "Magnetic Field Vector magnitude (T)":dbl=0.38999904300210686 format="%#_13g"
  in  "From 2":dbl[](array[numeric])=[0.15] min=-3000.0 max=3000.0 format="%#.5f"
  in  "To 2":dbl[](array[numeric])=[0.4] min=-3000.0 max=3000.0 format="%#.5g"
  in  "Step 2":dbl[](array[numeric])=[0.01] min=-3000.0 max=3000.0 format="%.3g"
  in  "Wait time after each sweep(min)":dbl format="%#_13g"
  out "Z-axis Magnetic Field (T)":string="0.330266838\r\n"
  in  "Y-axis Field ramp rate (T/min)":string="0.005"
  in  "Z-axis Field ramp rate (T/min)":string="0.005"
  out "Z-axis (90 deg)":dbl(slide)=0.330266838 scale=0.0..3.0
  out "Y-Axis (0deg)":dbl(slide)=-0.207420031 scale=0.0..3.0
  out "Y-axis Magnetic Field (T)":string="-0.207420031\r\n"
  in  "Magnet IP Address Z-axis":string="169.254.134.245"
  in  "Magnet IP Address Y-axis":string="169.254.212.113"
  in  "Magnetic field stabilization time (s)":dbl=2.0 format="%#_13g"
  in  "Step":dbl[](array[numeric])=[0.1] min=-3000.0 max=3000.0 format="%.4g"
  in  "To":dbl[](array[numeric])=[122.13] min=-3000.0 max=3000.0 format="%.4f"
  in  "From":dbl[](array[numeric])=[122.13] min=-3000.0 max=3000.0 format="%.4f"
  in  "Folder":path=path "D:/Pranava/Data/NiTe2/20-01-2021"
  in  "File name":string="006_NiTe2_13-12-2021_001_DeviceB_I_31-33_V_30-35_AC_IV(H)_with_second_harmonic_current_10Mohmbuffer_7.919Hz_7mK_150-400mT_122.13deg(perpendicular_to_current)_50ave_float"
  out "File path":path=path "D:/Pranava/Data/NiTe2/20-01-2021/006_NiTe2_13-12-2021_001_DeviceB_I_31-33_V_30-35_AC_IV(H)_with_second_harmonic_current_10Mohmbuffer_7.919Hz_7mK_150-400mT_122.13deg(perpendicular_to_current)_50ave_float.dat"
  # "Z-Axis: In-plane (90 deg)\nY-axis: Out-of-plane (0 deg)"
  # "[Must be less than 0.05]"
  # ".dat"
  # "It is important that there is enough time for the magnet to cool down after each sweep (Typically 15-20 min)"
  # "Configure Field magnitude (T)"
  # "Configure Field Angle (deg)"
  # "Configure MFLI voltage output (V)"
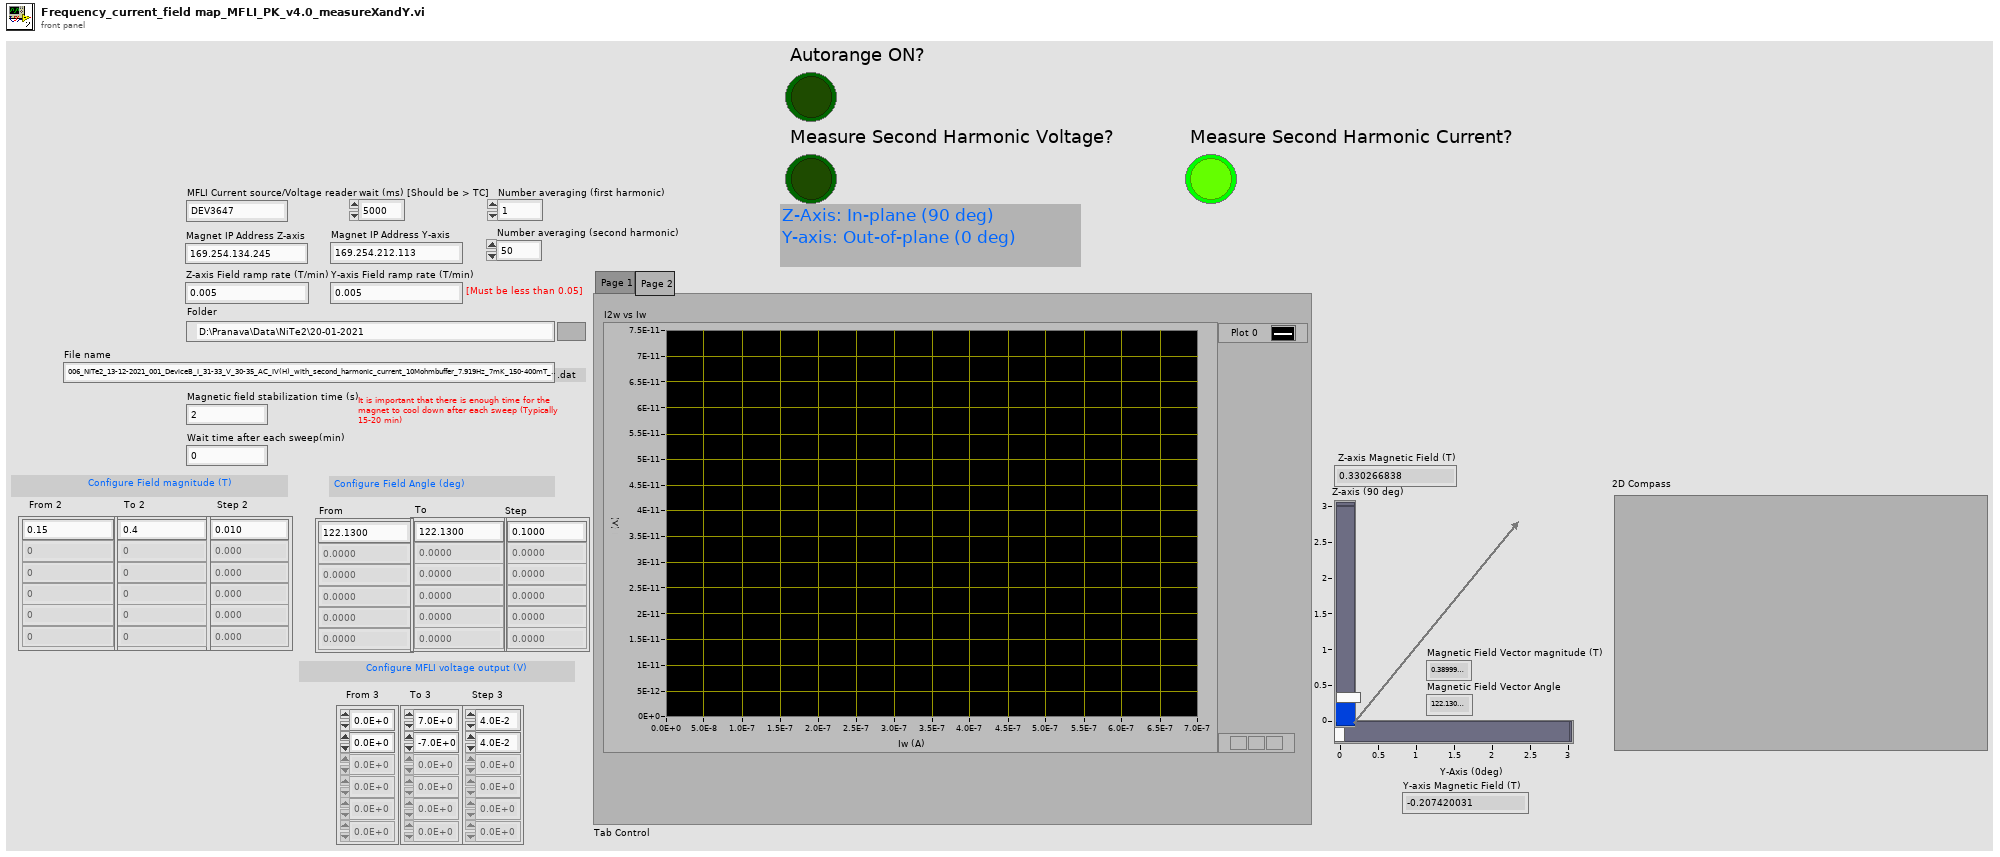
[diagram p1: front panel]
types:
  T1 = typedef "Zurich Instruments LabOne.lvlib/ziTypeHandle.ctl" = cluster{"handleValid":bool, "Conn":u64, "Path Prefix":string, "Handle":u64, "Connected":bool, "Clockbase(s)":dbl}
  T2 = enum16{"open", "replace", "create", "open or create", "replace or create", "replace or create with confirmation"}
  T3 = typedef "Zurich Instruments LabOne.lvlib/ziTypeDemodSampleSingle.ctl" = cluster{"Timestamps (ticks)":u64, "X (Vrms)":dbl, "Y (Vrms)":dbl, "Osc Phase (deg)":dbl, "Freq (Hz)":dbl, "DIO":u32, "AuxIn0 (V)":dbl, "AuxIn1 (V)":dbl, "Trigger":u32}
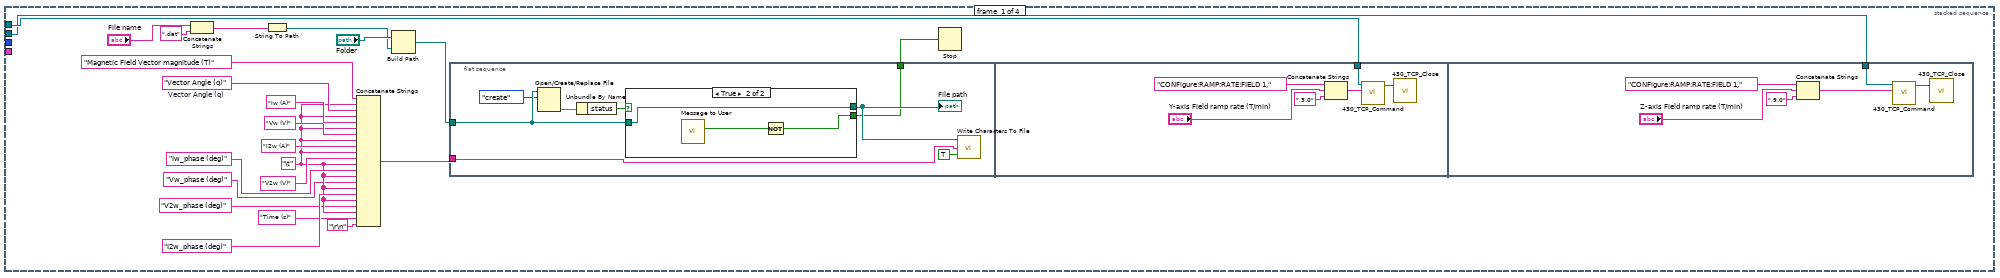
[diagram p2: hidden frame]
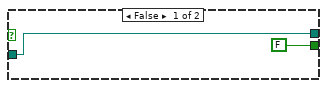
[diagram p3: hidden frame]
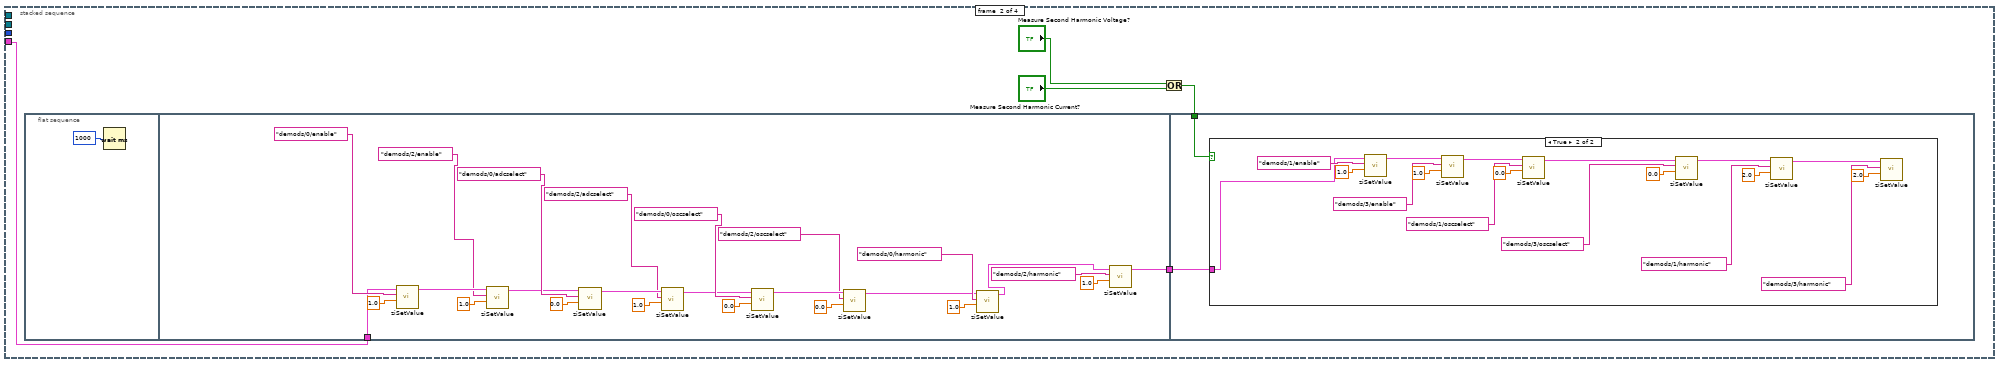
[diagram p4: hidden frame]
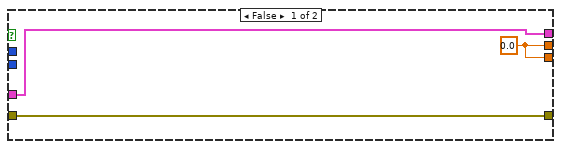
[diagram p8: hidden frame]
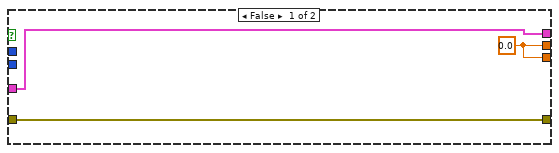
[diagram p9: hidden frame]
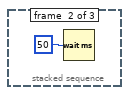
[diagram p10: hidden frame]
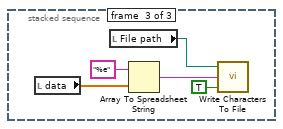
[diagram p11: hidden frame]
diagram:
  n1 = call "ziOpen.vi"("Address"="MFLI Current source/Voltage reader") -> ("Error Out"=w4:errorcluster, "HandleOut"=w5:T1)  [unwired: 3 in, 1 out]
  n2 = call "ziCheckVersion.vi"("Handle In"=w5, "Error In"=w4) -> ("Handle Out"=w2:T1)  [unwired: 11 in, 2 out]
  n3 = call "430_TCP_Open.vi"("IP Address"="Magnet IP Address Y-axis", "TCP Port"=7180) -> ("connection ID"=w11:refnum<k5>)  [unwired: 4 in, 2 out]
  n4 = call "430_TCP_Open.vi"("IP Address"="Magnet IP Address Z-axis", "TCP Port"=7180) -> ("connection ID"=w6:refnum<k5>)  [unwired: 4 in, 2 out]
  n5 = Tick Count (ms)() -> (millisecond timer value=w10:u32)
  n6 = stacked-sequence {
    tunnel: w11 -> [w26 _ _ _]
    tunnel: w10 -> [_ _ w117 _]
    tunnel: w6 -> [w24 _ _ _]
    tunnel: w2 -> [_ w65 w113 _]
    tunnel: [_ _ w112 _] -> w1
    frame #0 {
      w23 = "Vector Angle (q)"  # Vector Angle (q)
      w16 = "\t"
      n7 = Concatenate Strings("File name", ".dat" ("string")) -> (w33:string)
      n8 = String To Path(string=w33) -> (path=w28:path)
      n9 = Concatenate Strings("Magnetic Field Vector magnitude (T)", w16, w23, w16, "Iw (A)" ("string"), w16, "Vw (V)" ("string"), w16, "I2w (A)" ("string"), w16, "V2w (V)" ("string"), w16, "Iw_phase (deg)", w16, "Vw_phase (deg)", w16, "I2w_phase (deg)", w16, "V2w_phase (deg)", w16, "Time (s)", "\r\n") -> (w34:string)
      n10 = Build Path(base path="Folder", name or relative path=w28) -> (appended path=w27:path)
      n11 = flat-sequence {
        tunnel: [w40] -> w31
        tunnel: w34 -> [w42]
        tunnel: w27 -> [w39]
        tunnel: w26 -> [w50]
        tunnel: w24 -> [w55]
        frame #0 {
          n12 = Open/Create/Replace File(file path (use dialog)=w39, operation (0:open)=T2."create") -> (error out=w38:errorcluster)  [unwired: 4 in, 2 out]
          n13 = Unbundle By Name(w38) -> ("status"=w36:bool)
          n14 = case shown="True" w36 {
            tunnel: [FALSE ("Yes") w47] -> w40
            tunnel: [w44 w46] -> w41
            tunnel: w39 -> [w44 w46]
            frame False {
            }
            frame True {
              n15 = call "Message to User"() -> ("Yes"=w48:bool)  [unwired: 10 in, 1 out]
              n16 = Not(x=w48) -> (.not. x?=w47:bool)
            }
          }
          "File path" <- w41
          n17 = call <vilib>:"Write Characters To File.vi"("append to file? (new file:F)"=TRUE, "character string"=w42, "file path (dialog if empty)"=w41) -> ()  [unwired: 2 in, 1 out]
        }
        frame #1 {
          n18 = Concatenate Strings("CONFigure:RAMP:RATE:FIELD 1," ("String"), "Y-axis Field ramp rate (T/min)", ",3.0") -> (w51:string)
          n19 = call "430_TCP_Command.vi"("Command"=w51, "connection ID"=w50) -> ("connection ID out"=w54:refnum<k5>)  [unwired: 2 in, 2 out]
          n20 = call "430_TCP_Close.vi"("connection ID"=w54) -> ()  [unwired: 1 in, 2 out]
        }
        frame #2 {
          n21 = Concatenate Strings("CONFigure:RAMP:RATE:FIELD 1," ("String"), "Z-axis Field ramp rate (T/min)", ",9.0") -> (w57:string)
          n22 = call "430_TCP_Command.vi"("Command"=w57, "connection ID"=w55) -> ("connection ID out"=w60:refnum<k5>)  [unwired: 2 in, 2 out]
          n23 = call "430_TCP_Close.vi"("connection ID"=w60) -> ()  [unwired: 1 in, 2 out]
        }
      }
      n24 = Stop(stop? (T)=w31) -> ()
    }
    frame #1 {
      n25 = flat-sequence {
        tunnel: w65 -> [w67]
        tunnel: [w81] -> w64
        tunnel: w64 -> [w93]
        tunnel: w61 -> [w92]
        frame #0 {
          n26 = Wait (ms)(milliseconds to wait=u32 1000) -> ()  [unwired: 1 out]
        }
        frame #1 {
          n27 = call-poly "ziSetValue.vi"("Value"=1.0, "Path"="demods/0/enable", "Handle In"=w67) -> ("Handle Out"=w73:T1)  [unwired: 2 in, 1 out]
          n28 = call-poly "ziSetValue.vi"("Value"=1.0, "Path"="demods/2/enable", "Handle In"=w73) -> ("Handle Out"=w68:T1)  [unwired: 2 in, 1 out]
          n29 = call-poly "ziSetValue.vi"("Value"=0.0, "Path"="demods/0/adcselect", "Handle In"=w68) -> ("Handle Out"=w91:T1)  [unwired: 2 in, 1 out]
          n30 = call-poly "ziSetValue.vi"("Value"=1.0, "Path"="demods/2/adcselect", "Handle In"=w91) -> ("Handle Out"=w75:T1)  [unwired: 2 in, 1 out]
          n31 = call-poly "ziSetValue.vi"("Value"=0.0, "Path"="demods/0/oscselect", "Handle In"=w75) -> ("Handle Out"=w80:T1)  [unwired: 2 in, 1 out]
          n32 = call-poly "ziSetValue.vi"("Value"=0.0, "Path"="demods/2/oscselect", "Handle In"=w80) -> ("Handle Out"=w74:T1)  [unwired: 2 in, 1 out]
          n33 = call-poly "ziSetValue.vi"("Value"=1.0, "Path"="demods/0/harmonic", "Handle In"=w74) -> ("Handle Out"=w86:T1)  [unwired: 2 in, 1 out]
          n34 = call-poly "ziSetValue.vi"("Value"=1.0, "Path"="demods/2/harmonic", "Handle In"=w86) -> ("Handle Out"=w81:T1)  [unwired: 2 in, 1 out]
        }
        frame #2 {
          n35 = case shown="True" w92 {
            tunnel: w93 -> [_ w101]
            frame False {
            }
            frame True {
              n36 = call-poly "ziSetValue.vi"("Value"=1.0, "Path"="demods/1/enable", "Handle In"=w101) -> ("Handle Out"=w106:T1)  [unwired: 2 in, 1 out]
              n37 = call-poly "ziSetValue.vi"("Value"=1.0, "Path"="demods/3/enable", "Handle In"=w106) -> ("Handle Out"=w95:T1)  [unwired: 2 in, 1 out]
              n38 = call-poly "ziSetValue.vi"("Value"=0.0, "Path"="demods/1/oscselect", "Handle In"=w95) -> ("Handle Out"=w100:T1)  [unwired: 2 in, 1 out]
              n39 = call-poly "ziSetValue.vi"("Value"=0.0, "Path"="demods/3/oscselect", "Handle In"=w100) -> ("Handle Out"=w94:T1)  [unwired: 2 in, 1 out]
              n40 = call-poly "ziSetValue.vi"("Value"=2.0, "Path"="demods/1/harmonic", "Handle In"=w94) -> ("Handle Out"=w111:T1)  [unwired: 2 in, 1 out]
              n41 = call-poly "ziSetValue.vi"("Value"=2.0, "Path"="demods/3/harmonic", "Handle In"=w111) -> ()  [unwired: 2 in, 2 out]
            }
          }
        }
      }
      n42 = Or(x="Measure Second Harmonic Voltage?", y="Measure Second Harmonic Current?") -> (x .or. y?=w61:bool)
    }
    frame #2 {
      n43 = for {
        tunnel: w117 -> [w124]
        tunnel: "From 2" -> [w123] mode=indexing
        tunnel: "To 2" -> [w122] mode=indexing
        tunnel: "Step 2" -> [w121] mode=indexing
        shift-right: [w118] -> w112
        shift-left: w113 -> [w119]
        n44 = call "Build_serie_EL.vi"("end value"=w122, "increment"=w121, "start value"=w123) -> ("output array"=w120:dbl[])
        n45 = for {
          tunnel: w124 -> [w128]
          tunnel: w120 -> [w127] mode=indexing
          shift-right: [w125] -> w118
          shift-left: w119 -> [w126]
          n46 = for {
            tunnel: "From" -> [w143] mode=indexing
            tunnel: "To" -> [w141] mode=indexing
            tunnel: "Step" -> [w142] mode=indexing
            tunnel: w128 -> [w140]
            tunnel: w127 -> [w135]
            shift-right: [w132] -> w125
            shift-left: w126 -> [w133]
            n47 = flat-sequence {
              tunnel: w140 -> [w145]
              tunnel: w141 -> [w146]
              tunnel: w142 -> [w147]
              tunnel: w143 -> [w148]
              tunnel: [w148] -> w139
              tunnel: [w147] -> w138
              tunnel: [w146] -> w137
              tunnel: [w145] -> w136
              tunnel: w135 -> [w144]
              tunnel: [w144] -> w134
              tunnel: w139 -> [w156]
              tunnel: w138 -> [w155]
              tunnel: w137 -> [w154]
              tunnel: w136 -> [w152]
              tunnel: w134 -> [w151]
              tunnel: w133 -> [w150]
              tunnel: [w149] -> w132
              frame #0 {
              }
              frame #1 {
                n48 = call "Build_serie_EL.vi"("end value"=w154, "increment"=w155, "start value"=w156) -> ("output array"=w153:dbl[])
                n49 = for {
                  tunnel: w153 -> [w165] mode=indexing
                  tunnel: w152 -> [w159]
                  tunnel: w151 -> [w164]
                  shift-right: [w157] -> w149
                  shift-left: w150 -> [w158]
                  n50 = flat-sequence {
                    tunnel: [w168] -> w163
                    tunnel: [w169] -> w160
                    tunnel: w164 -> [w166]
                    tunnel: w165 -> [w167]
                    tunnel: w163 -> [w182]
                    tunnel: [w182] -> w162
                    tunnel: [w181] -> w161
                    tunnel: w160 -> [w181]
                    tunnel: w161 -> [_]
                    tunnel: w162 -> [_]
                    tunnel: w159 -> [w193]
                    tunnel: w158 -> [w187]
                    tunnel: [w186] -> w157
                    frame #0 {
                      n51 = local read "Z-axis Field ramp rate (T/min)"() -> (w177:string)
                      n52 = local read "Y-axis Field ramp rate (T/min)"() -> (w178:string)
                      n53 = local read "Magnet IP Address Z-axis"() -> (w180:string)
                      n54 = local read "Magnet IP Address Y-axis"() -> (w179:string)
                      n55 = call "Set2D_Magneticfield(polar)_PK.vi"("Y-axis Ramp Rate (T/min)"=w178, "Z-axis Ramp Rate (T/min)"=w177, "Set target vector angle (degrees)"=w167, "Set target vector magnitude (T)"=w166, "Y-Axis Magnet IP Address"=w179, "Z-Axis Magnet IP Address"=w180) -> ("Z-axis Magnetic Field (T)"=w174:string, "Y-axis Magnetic Field (T)"=w176:string, "q - Vector angle"=w169:dbl, "R - Vector field magnitude (T)"=w168:dbl)  [unwired: 2 in]
                      "Z-axis Magnetic Field (T)" <- w174
                      "Y-axis Magnetic Field (T)" <- w176
                      "Magnetic Field Vector magnitude (T)" <- w168
                      "Magnetic Field Vector Angle" <- w169
                      n56 = Fract/Exp String To Number(string=w176) -> (number=→"Y-Axis (0deg)":dbl)  [unwired: 3 in, 1 out]
                      n57 = Fract/Exp String To Number(string=w174) -> (number=→"Z-axis (90 deg)":dbl)  [unwired: 3 in, 1 out]
                      n58 = Build Array(w169) -> (w170:dbl[])
                      n59 = Build Array(w168) -> (w171:dbl[])
                      n60 = call-poly <vilib>:"Plot Helper.vi"("radius vector"=w171, "theta vector"=w170) -> ("2D Plot Class Obj Array out"=→"2D Compass":refnum<class "2D Plot Datatype.lvclass">[])  [unwired: 2 in, 7 out]
                    }
                    frame #1 {
                      n61 = Multiply(x="Magnetic field stabilization time (s)", y=1000) -> (x*y=w184:dbl)
                      n62 = Wait (ms)(milliseconds to wait=w184) -> ()  [unwired: 1 out]
                    }
                    frame #2 {
                      n63 = for {
                        tunnel: "From 3" -> [w203] mode=indexing
                        tunnel: "To 3" -> [w202] mode=indexing
                        tunnel: "Step 3" -> [w201] mode=indexing
                        shift-right: [w205] -> _
                        shift-left: cluster{dbl, "Field Reading":dbl}[] [] -> [w206]
                        tunnel: w193 -> [w200]
                        shift-right: [w199] -> _
                        shift-left: cluster{dbl, "Field Reading":dbl}[] [] -> [w198]
                        shift-right: [w197] -> w186
                        shift-left: w187 -> [w195]
                        shift-right: [w196] -> _
                        shift-left: _ -> [w194]
                        n64 = call "Build_serie_EL.vi"("end value"=w202, "increment"=w201, "start value"=w203) -> ("output array"=w204:dbl[])
                        n65 = for {
                          tunnel: w204 -> [w221] mode=indexing
                          shift-right: [w219] -> w205
                          shift-left: w206 -> [w220]
                          shift-right: [w216] -> w197
                          shift-left: w195 -> [w218]
                          shift-right: [w215] -> w196
                          shift-left: w194 -> [w217]
                          tunnel: w200 -> [w211]
                          shift-right: [w209] -> w199
                          shift-left: w198 -> [w208]
                          i -> [w207]
                          n66 = Tick Count (ms)() -> (millisecond timer value=w212:u32)
                          n67 = Subtract(x=w212, y=w211) -> (x-y=w213:u32)
                          n68 = Divide(x=w213, y=1000) -> (x/y=w210:dbl)
                          "Time(s)" <- w210
                          n69 = stacked-sequence {
                            tunnel: w221 -> [w253 _ _]
                            tunnel: w220 -> [w254 _ _]
                            tunnel: [w255 _ _] -> w219
                            tunnel: w218 -> [w252 _ _]
                            tunnel: w217 -> [w251 _ _]
                            tunnel: [w247 _ _] -> w216
                            tunnel: [w246 _ _] -> w215
                            tunnel: w210 -> [_ _ _]
                            tunnel: [w233 _ _] -> w209
                            tunnel: w208 -> [w232 _ _]
                            tunnel: w207 -> [w225 _ _]
                            frame #0 {
                              n70 = flat-sequence {
                                tunnel: [w270] -> w231
                                tunnel: w253 -> [w269]
                                tunnel: w254 -> [w270]
                                tunnel: [w258] -> w229
                                tunnel: [w259] -> w227
                                tunnel: w252 -> [w261]
                                tunnel: w251 -> [w260]
                                tunnel: w231 -> [w287]
                                tunnel: [w287] -> w230
                                tunnel: w229 -> [w286]
                                tunnel: [w286] -> w228
                                tunnel: w227 -> [w285]
                                tunnel: [w285] -> w226
                                tunnel: w225 -> [w283]
                                tunnel: w230 -> [w292]
                                tunnel: [w292] -> w222
                                tunnel: [w290] -> w223
                                tunnel: [w289] -> w224
                                tunnel: w228 -> [w289]
                                tunnel: w226 -> [w290]
                                tunnel: [w304] -> w250
                                tunnel: [w301] -> w249
                                tunnel: [w300] -> w248
                                tunnel: ["Number averaging (first harmonic)"] -> w238
                                tunnel: w222 -> [w304]
                                tunnel: w223 -> [w302]
                                tunnel: w224 -> [w303]
                                tunnel: w250 -> [w326]
                                tunnel: [w326] -> w245
                                tunnel: w249 -> [w325]
                                tunnel: w248 -> [w324]
                                tunnel: [w323] -> w244
                                tunnel: [w322] -> w243
                                tunnel: w238 -> [w315]
                                tunnel: w245 -> [w345]
                                tunnel: [w345] -> w242
                                tunnel: w244 -> [w344]
                                tunnel: w243 -> [w343]
                                tunnel: [w341] -> w240
                                tunnel: [w342] -> w237
                                tunnel: ["Number averaging (second harmonic)"] -> w235
                                tunnel: ["Number averaging (second harmonic)"] -> w234
                                tunnel: w242 -> [w380]
                                tunnel: [w380] -> w241
                                tunnel: w240 -> [w378]
                                tunnel: [w376] -> w239
                                tunnel: w237 -> [w379]
                                tunnel: [w377] -> w236
                                tunnel: w235 -> [w375]
                                tunnel: w234 -> [w374]
                                tunnel: [w424] -> w255
                                tunnel: w241 -> [w423]
                                tunnel: [w422] -> w247
                                tunnel: [w421] -> w246
                                tunnel: w239 -> [w421]
                                tunnel: w236 -> [w422]
                                tunnel: [w418] -> w233
                                tunnel: w232 -> [w417]
                                frame #0 {
                                n71 = Square Root(x=2.0) -> (sqrt(x)=w268:dbl)
                                n72 = Multiply(x=w269, y=w268) -> (x*y=w257:dbl)
                                "Set Voltage(V)" <- w257
                                n73 = call-poly "ziSetValue.vi"("Error In"=w260, "Value"=w257, "Path"="sigouts/0/amplitudes/0", "Handle In"=w261) -> ("Error Out"=w264:errorcluster, "Handle Out"=w265:T1)  [unwired: 1 in]
                                n74 = case shown="True" "Autorange ON?" {
                                tunnel: w265 -> [w272 w282]
                                tunnel: w264 -> [w271 w279]
                                tunnel: [w272 w274] -> w263
                                tunnel: [w271 w273] -> w262
                                frame False {
                                }
                                frame True {
                                n75 = call-poly "ziSetValue.vi"("Error In"=w279, "Value"=1.0, "Path"="sigins/0/autorange", "Handle In"=w282) -> ("Error Out"=w275:errorcluster, "Handle Out"=w276:T1)  [unwired: 1 in]
                                n76 = call-poly "ziSetValue.vi"("Error In"=w275, "Value"=1.0, "Path"="currins/0/autorange", "Handle In"=w276) -> ("Error Out"=w273:errorcluster, "Handle Out"=w274:T1)  [unwired: 1 in]
                                }
                                }
                                n77 = call "ziSync.vi"("Handle In"=w263, "Error In"=w262) -> ("Handle Out"=w259:T1, "Error Out"=w258:errorcluster)  [unwired: 12 in]
                                }
                                frame #1 {
                                n78 = Equal To 0?(x=w283) -> (x = 0?=w284:bool)
                                n79 = case shown="True" w284 {
                                frame False {
                                }
                                frame True {
                                n80 = Wait (ms)(milliseconds to wait=10000) -> ()  [unwired: 1 out]
                                }
                                }
                                }
                                frame #2 {
                                n81 = Wait (ms)(milliseconds to wait="wait (ms) [Should be > TC]") -> ()  [unwired: 1 out]
                                }
                                frame #3 {
                                n82 = for {
                                N: "Number averaging (first harmonic)" -> [_]
                                tunnel: [w306] -> w296 mode=indexing
                                tunnel: [w305] -> w294 mode=indexing
                                shift-right: [w309] -> w300
                                shift-left: w303 -> [w312]
                                shift-right: [w310] -> w301
                                shift-left: w302 -> [w311]
                                n83 = call-poly "ziGetValue.vi"("error in"=w312, "Path"="demods/0/sample", "Handle In"=w311) -> ("error out"=w309:errorcluster, "Demod Sample Out"=w313:T3, "Handle Out"=w310:T1)
                                n84 = Unbundle By Name(w313) -> ("X (Vrms)"=w308:dbl, "Y (Vrms)"=w307:dbl)
                                n85 = Re/Im To Polar(2:w307, 3:w308) -> (0:w305:dbl, 1:w306:dbl)
                                }
                                n86 = call "Array averaging_PK.vi"("Number averaging"="Number averaging (first harmonic)", "numeric array"=w296) -> ("Average value"=→"Vw (V)":dbl)  [unwired: 9 in]
                                n87 = call "Array averaging_PK.vi"("Number averaging"="Number averaging (first harmonic)", "numeric array"=w294) -> ("Average value"=w295:dbl)  [unwired: 9 in]
                                n88 = Multiply(x=w295, y=57.28835136855506) -> (x*y=→"Vw_phase (deg)":dbl)
                                }
                                frame #4 {
                                n89 = for {
                                N: w315 -> [_]
                                tunnel: [w328] -> w317 mode=indexing
                                tunnel: [w327] -> w316 mode=indexing
                                shift-right: [w332] -> w323
                                shift-left: w325 -> [w334]
                                shift-right: [w331] -> w322
                                shift-left: w324 -> [w333]
                                n90 = call-poly "ziGetValue.vi"("error in"=w333, "Path"="demods/2/sample", "Handle In"=w334) -> ("error out"=w331:errorcluster, "Demod Sample Out"=w335:T3, "Handle Out"=w332:T1)
                                n91 = Unbundle By Name(w335) -> ("X (Vrms)"=w329:dbl, "Y (Vrms)"=w330:dbl)
                                n92 = Re/Im To Polar(2:w330, 3:w329) -> (0:w327:dbl, 1:w328:dbl)
                                }
                                n93 = call "Array averaging_PK.vi"("Number averaging"=w315, "numeric array"=w317) -> ("Average value"=→"Iw (A)":dbl)  [unwired: 9 in]
                                n94 = call "Array averaging_PK.vi"("Number averaging"=w315, "numeric array"=w316) -> ("Average value"=w318:dbl)  [unwired: 9 in]
                                n95 = Multiply(x=w318, y=57.28835136855506) -> (x*y=→"Iw_phase (deg)":dbl)
                                }
                                frame #5 {
                                n96 = local read "Measure Second Harmonic Voltage?"() -> (w338:bool)
                                n97 = case shown="True" w338 {
                                tunnel: w344 -> [w348 w359]
                                tunnel: w343 -> [w347 w358]
                                tunnel: [w348 w354] -> w342
                                tunnel: [w347 w353] -> w341
                                tunnel: "Number averaging (second harmonic)" -> [_ w352]
                                tunnel: "Number averaging (second harmonic)" -> [_ w351]
                                tunnel: [w346 w350] -> w340
                                tunnel: [w346 w349] -> w339
                                frame False {
                                w346 = 0.0
                                }
                                frame True {
                                n98 = for {
                                N: w352 -> [_]
                                tunnel: [w366] -> w355 mode=indexing
                                tunnel: [w365] -> w357 mode=indexing
                                shift-right: [w362] -> w354
                                shift-left: w359 -> [w364]
                                shift-right: [w361] -> w353
                                shift-left: w358 -> [w363]
                                n99 = call-poly "ziGetValue.vi"("error in"=w363, "Path"="demods/1/sample", "Handle In"=w364) -> ("error out"=w361:errorcluster, "Demod Sample Out"=w369:T3, "Handle Out"=w362:T1)
                                n100 = Unbundle By Name(w369) -> ("X (Vrms)"=w368:dbl, "Y (Vrms)"=w367:dbl)
                                n101 = Re/Im To Polar(2:w367, 3:w368) -> (0:w365:dbl, 1:w366:dbl)
                                }
                                n102 = call "Array averaging_PK.vi"("Number averaging"=w351, "numeric array"=w355) -> ("Average value"=w350:dbl)  [unwired: 9 in]
                                n103 = call "Array averaging_PK.vi"("Number averaging"=w351, "numeric array"=w357) -> ("Average value"=w356:dbl)  [unwired: 9 in]
                                n104 = Multiply(x=w356, y=57.28835136855506) -> (x*y=w349:dbl)
                                }
                                }
                                "V2w (V)" <- w340
                                "V2w_phase (deg)" <- w339
                                }
                                frame #6 {
                                n105 = local read "Measure Second Harmonic Current?"() -> (w371:bool)
                                n106 = case shown="True" w371 {
                                tunnel: w379 -> [w383 w394]
                                tunnel: w378 -> [w382 w393]
                                tunnel: [w383 w392] -> w377
                                tunnel: [w382 w391] -> w376
                                tunnel: w375 -> [_ w387]
                                tunnel: w374 -> [_ w386]
                                tunnel: [w381 w385] -> w373
                                tunnel: [w381 w384] -> w372
                                frame False {
                                w381 = 0.0
                                }
                                frame True {
                                n107 = for {
                                N: w387 -> [_]
                                tunnel: [w401] -> w390 mode=indexing
                                tunnel: [w400] -> w388 mode=indexing
                                shift-right: [w397] -> w392
                                shift-left: w394 -> [w399]
                                shift-right: [w396] -> w391
                                shift-left: w393 -> [w398]
                                n108 = call-poly "ziGetValue.vi"("error in"=w398, "Path"="demods/3/sample", "Handle In"=w399) -> ("error out"=w396:errorcluster, "Demod Sample Out"=w404:T3, "Handle Out"=w397:T1)
                                n109 = Unbundle By Name(w404) -> ("X (Vrms)"=w403:dbl, "Y (Vrms)"=w402:dbl)
                                n110 = Re/Im To Polar(2:w402, 3:w403) -> (0:w400:dbl, 1:w401:dbl)
                                }
                                n111 = call "Array averaging_PK.vi"("Number averaging"=w386, "numeric array"=w390) -> ("Average value"=w385:dbl)  [unwired: 9 in]
                                n112 = call "Array averaging_PK.vi"("Number averaging"=w386, "numeric array"=w388) -> ("Average value"=w389:dbl)  [unwired: 9 in]
                                n113 = Multiply(x=w389, y=57.28835136855506) -> (x*y=w384:dbl)
                                }
                                }
                                "I2w (A)" <- w373
                                "I2w_phase (deg)" <- w372
                                }
                                frame #7 {
                                n114 = local read "Magnetic Field Vector magnitude (T)"() -> (w416:dbl)
                                n115 = local read "Magnetic Field Vector Angle"() -> (w415:dbl)
                                n116 = local read "I2w (A)"() -> (w412:dbl)
                                n117 = local read "Vw (V)"() -> (w413:dbl)
                                n118 = local read "Iw (A)"() -> (w414:dbl)
                                n119 = local read "V2w_phase (deg)"() -> (w407:dbl)
                                n120 = local read "I2w_phase (deg)"() -> (w408:dbl)
                                n121 = local read "Vw_phase (deg)"() -> (w410:dbl)
                                n122 = local read "Iw_phase (deg)"() -> (w409:dbl)
                                n123 = local read "V2w (V)"() -> (w411:dbl)
                                n124 = local read "Time(s)"() -> (w406:dbl)
                                n125 = Bundle("Iw (A)"=w414, "Vw (V)"=w413) -> (w420:cluster{"Iw (A)":dbl, "Vw (V)":dbl})  [unwired: 1 in]
                                n126 = Bundle("Iw (A)"=w414, "I2w (A)"=w412) -> (w419:cluster{"Iw (A)":dbl, "I2w (A)":dbl})  [unwired: 1 in]
                                n127 = Build Array (concatenate)(w423, w420) -> (w424:cluster{"Iw (A)":dbl, "Vw (V)":dbl}[])
                                "Iw vs Vw" <- w424
                                n128 = Build Array (concatenate)(w417, w419) -> (w418:cluster{"Iw (A)":dbl, "I2w (A)":dbl}[])
                                "I2w vs Iw" <- w418
                                n129 = Build Array(w416, w415, w414, w413, w412, w411, w409, w410, w408, w407, w406) -> (→"data":dbl[])
                                }
                              }
                            }
                            frame #1 {
                              n130 = Wait (ms)(milliseconds to wait=u32 50) -> ()  [unwired: 1 out]
                            }
                            frame #2 {
                              n131 = local read "data"() -> (w428:dbl[])
                              n132 = local read "File path"() -> (w427:path)
                              n133 = Array To Spreadsheet String(array=w428, 3:"%e" ("format string")) -> (spreadsheet string=w430:string)  [unwired: 1 in]
                              n134 = call <vilib>:"Write Characters To File.vi"("append to file? (new file:F)"=TRUE, "character string"=w430, "file path (dialog if empty)"=w427) -> ()  [unwired: 2 in, 1 out]
                            }
                          }
                        }
                      }
                    }
                  }
                }
              }
              frame #2 {
                n135 = Multiply(x="Wait time after each sweep(min)", y=60000.0) -> (x*y=w434:dbl)
                n136 = Wait (ms)(milliseconds to wait=w434) -> ()  [unwired: 1 out]
              }
            }
          }
        }
      }
    }
    frame #3 {
    }
  }
  n137 = call "ziClose.vi"("Handle In"=w1) -> ()  [unwired: 1 in, 4 out]
